vi "Navx data.vi"() -> ()   [LabVIEW 2014]
uses:
  navx-mxp/roborio/labview/navX-MXP Library/COMMON/TypeDefs/Data TypeDefs/navX YPRH Data.ctl
  navx-mxp/roborio/labview/navX-MXP Library/navX-MXP IMU.lvlib
panel:
  out "Yaw Zero":dbl
  out "YPRH":T1
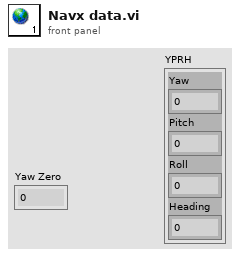
[diagram p1: front panel]
types:
  T1 = typedef "navX-MXP IMU.lvlib/navX YPRH Data.ctl" = cluster{"Yaw":dbl, "Pitch":dbl, "Roll":dbl, "Heading":dbl}
diagram:
